vi "Get Steps Array.vi"(8 "Error In":errorcluster, 11 "reference in":refnum<class "Recipe.lvclass">) -> (0 "Error Out":errorcluster, 2 "Steps":cluster{"Fire (%)":dbl, "Duration (s)":dbl}[](array[cluster]), 3 "reference out":refnum<class "Recipe.lvclass">)   [LabVIEW 2021, in "Recipe.lvclass"]
uses:
  Recipe.lvclass
  Recipe Step/Recipe Step.lvclass
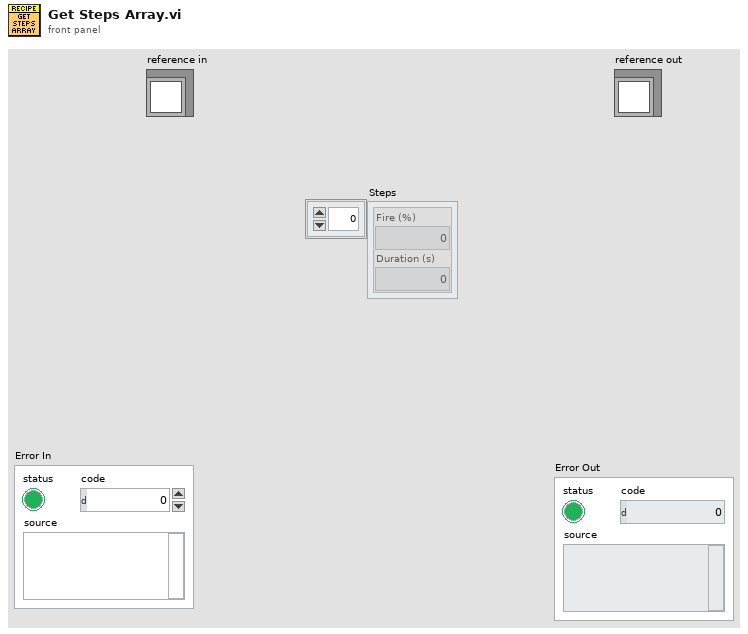
[diagram p1: front panel]
types:
  T1 = typedef "Recipe.lvclass/ObjectAttributes.ctl" = cluster{"Steps":refnum<class "Recipe Step.lvclass">[], "Current Info":cluster{"Current Index":u64}}
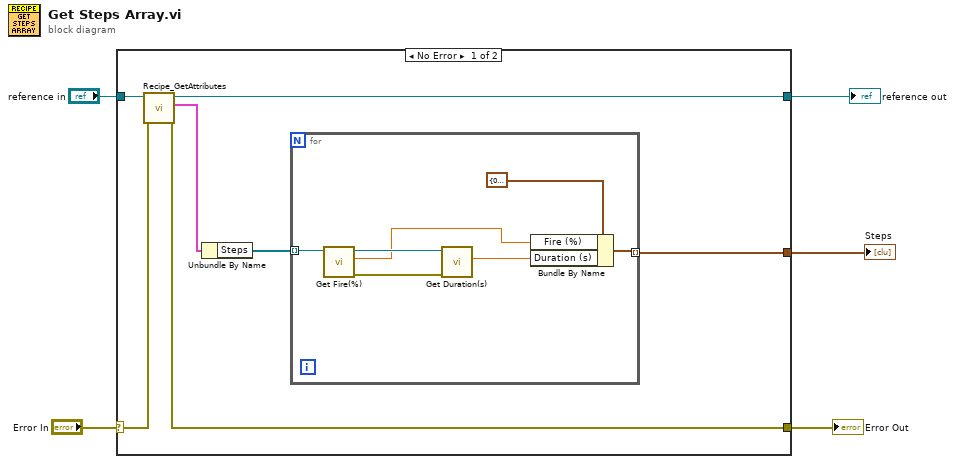
[diagram p0: block diagram]
diagram:
  n1 = case shown="No Error" "Error In" {
    selector: "Error In" -> [w12 w21]
    tunnel: [w10 w21] -> w4
    tunnel: [w8 w20] -> w2
    tunnel: "reference in" -> [w9 w20]
    tunnel: [w6 _] -> w1
    frame No Error {
      n2 = call "Recipe_GetAttributes.vi"("Error In"=w12, "reference in"=w9) -> ("Error Out"=w10:errorcluster, "Data"=w11:T1, "reference out"=w8:refnum<class "Recipe.lvclass">)  [unwired: 6 in, 1 out]
      n3 = Unbundle By Name(w11) -> ("Steps"=w7:refnum<class "Recipe Step.lvclass">[])
      n4 = for {
        tunnel: w7 -> [w19] mode=indexing
        tunnel: [w13] -> w6 mode=indexing
        n5 = call-dynamic "Get Fire(%).vi"("reference in"=w19) -> ("Error Out"=w18:errorcluster, "Fire (%)"=w15:dbl, "reference out"=w17:refnum<class "Recipe Step.lvclass">)  [unwired: 8 in]
        n6 = call-dynamic "Get Duration(s).vi"("Error In"=w18, "reference in"=w17) -> ("Duration (s)"=w14:dbl)  [unwired: 7 in, 2 out]
        n7 = Bundle By Name(cluster=cluster{"Fire (%)":dbl, "Duration (s)":dbl} {"Fire (%)"=0.0, "Duration (s)"=0.0} ("Data"), "Fire (%)"=w15, "Duration (s)"=w14) -> (w13:cluster{"Fire (%)":dbl, "Duration (s)":dbl})
      }
    }
    frame Error {
    }
  }
  "Error Out" <- w4
  "reference out" <- w2
  "Steps" <- w1
